vi "Update Drawing.vi"(8 "error in (no error)":errorcluster, 10 "Field Drawing":picture, 11 "Phoenix in":refnum<class "Phoenix.lvclass">) -> (0 "error out":errorcluster, 3 "Phoenix out":refnum<class "Phoenix.lvclass">)   [LabVIEW 2022 SP3, in "Phoenix.lvlib" / "Phoenix.lvclass"]
uses:
  Phoenix.lvclass
  Phoenix.lvclass/Phoenix.ctl
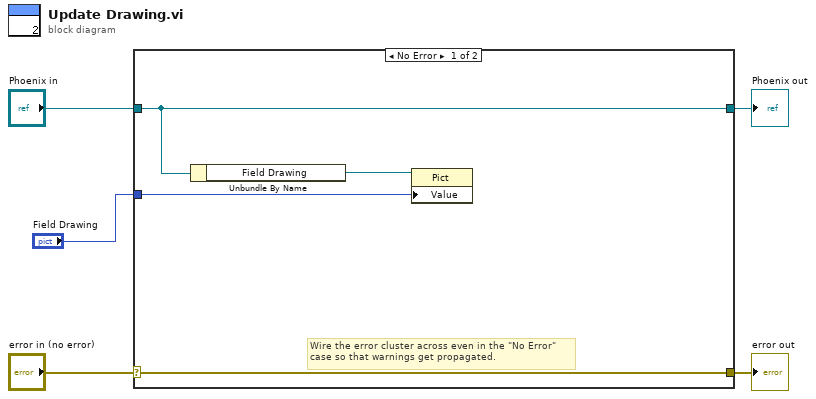
[diagram p0: block diagram]
diagram:
  n1 = case shown="No Error" "error in (no error)" {
    selector: "error in (no error)" -> [w9 w11]
    tunnel: [w9 w11] -> w4
    tunnel: [w8 w10] -> w2
    tunnel: "Phoenix in" -> [w8 w10]
    tunnel: "Field Drawing" -> [w6 _]
    frame No Error {
      # "Wire the error cluster across even in the \"No Error\"\ncase so that warnings get propagated."
      n2 = Unbundle By Name(w8) -> ("Field Drawing"=w7:refnum<vi>)
      n3 = property class="Pict"(reference=w7, "Value"=w6) -> ()  [unwired: 1 in, 2 out]
    }
    frame Error {
    }
  }
  "error out" <- w4
  "Phoenix out" <- w2
